vi "01_init.vi"(11 "COM port":refnum<visa-resource-name>) -> (1 "Data queue":refnum<queue>, 2 "outCMD queue":refnum<queue>, 3 "VISA resource name out":refnum<visa-resource-name>)   [LabVIEW 2017]
uses:
  <vilib>/Instr/_visa.llb/VISA Configure Serial Port (Instr).vi
panel:
  out "queue out":refnum<queue>
  out "CMDforData":refnum<queue>
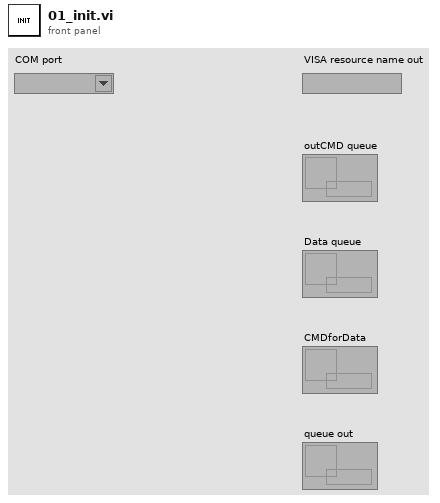
[diagram p1: front panel]
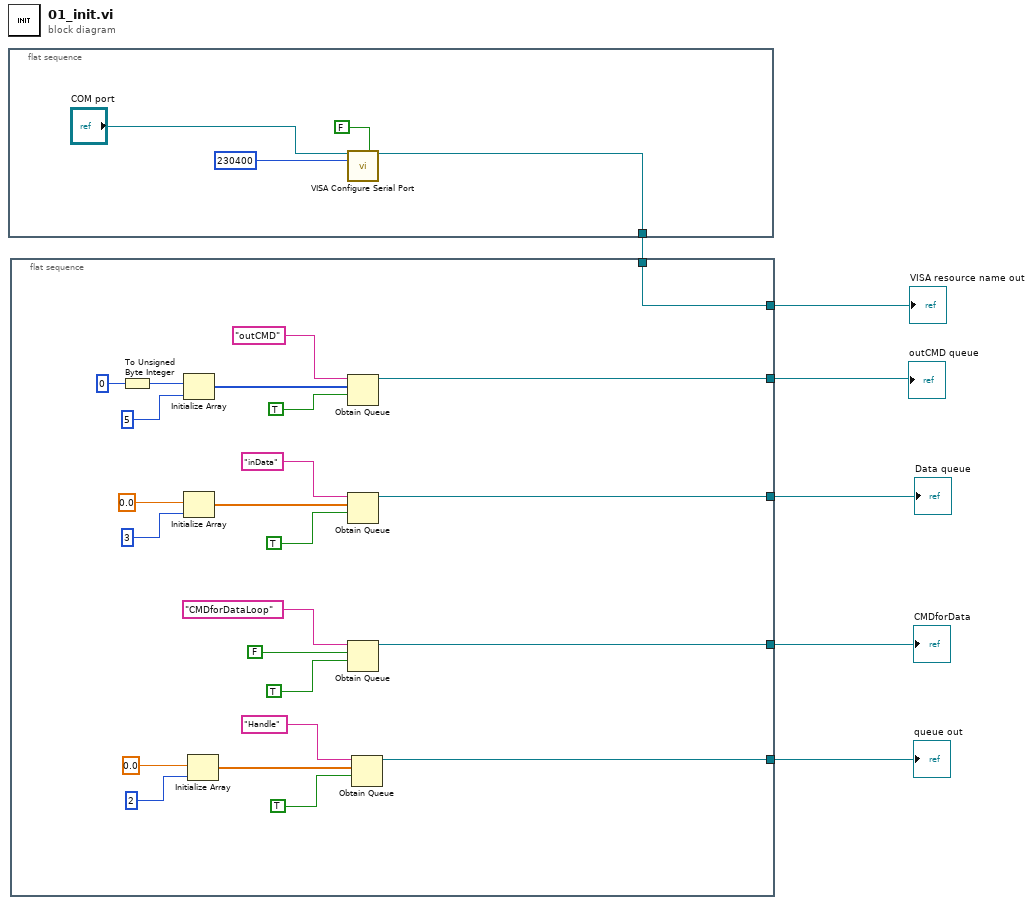
[diagram p0: block diagram]
diagram:
  n1 = flat-sequence {
    tunnel: [w7] -> w4
    frame #0 {
      n2 = call-poly "VISA Configure Serial Port"("VISA resource name"="COM port", "Enable Termination\nChar (T)"=FALSE ("Enable Termination\nChar (T)"), "baud rate (9600)"=u32 230400) -> ("VISA resource name out"=w7:refnum<visa-resource-name>)  [unwired: 11 in, 1 out]
    }
  }
  n3 = flat-sequence {
    tunnel: [w24] -> w3
    tunnel: [w23] -> w6
    tunnel: [w22] -> w5
    tunnel: w4 -> [w22]
    tunnel: [w17] -> w2
    tunnel: [w11] -> w1
    frame #0 {
      n4 = To Unsigned Byte Integer(number=u8 0) -> (unsigned 8bit integer=w34:u8)
      n5 = Initialize Array(w34, 5 ("dimension size")) -> (w31:u8[])
      n6 = Initialize Array(0.0, 3 ("dimension size")) -> (w26:dbl[])
      n7 = Initialize Array(0.0, 2 ("dimension size")) -> (w14:dbl[])
      n8 = Obtain Queue(name (unnamed)="outCMD", element data type=w31, create if not found? (T)=TRUE) -> (queue out=w23:refnum<queue>)  [unwired: 2 in, 2 out]
      n9 = Obtain Queue(name (unnamed)="inData", element data type=w26, create if not found? (T)=TRUE) -> (queue out=w24:refnum<queue>)  [unwired: 2 in, 2 out]
      n10 = Obtain Queue(name (unnamed)="CMDforDataLoop", element data type=FALSE ("create if not found? (T)"), create if not found? (T)=TRUE) -> (queue out=w17:refnum<queue>)  [unwired: 2 in, 2 out]
      n11 = Obtain Queue(name (unnamed)="Handle", element data type=w14, create if not found? (T)=TRUE) -> (queue out=w11:refnum<queue>)  [unwired: 2 in, 2 out]
    }
  }
  "outCMD queue" <- w6
  "VISA resource name out" <- w5
  "Data queue" <- w3
  "CMDforData" <- w2
  "queue out" <- w1
